vi "mqttCmdPublishAckCommand.vi"(9 "messageID":u16, 11 "error in (no error)":errorcluster) -> (15 "error out":errorcluster)   [LabVIEW 2015]
uses:
  mqttTypedef/mqttMessageType.ctl
  mqttTypedef/mqttQOSlevel.ctl
  mqttCmd.lvclass
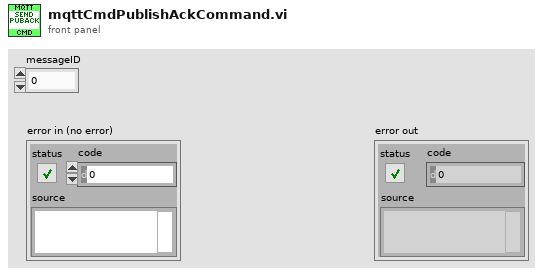
[diagram p1: front panel]
types:
  T1 = typedef "mqttQOSlevel.ctl" = enum8{"At most once", "At least once", "Exactly once", "Reserved"}
  T2 = typedef "mqttMessageType.ctl" = enum32{"Reserved", "CONNECT", "CONNACK", "PUBLISH", "PUBACK", "PUBREC", "PUBREL", "PUBCOMP", "SUBSCRIBE", "SUBACK", "UNSUBSCRIBE", "UNSUBACK", "PINGREQ", "PINGRESP", "DISCONNECT", "Reserved2"}
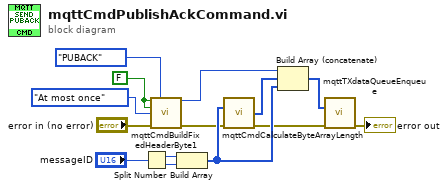
[diagram p0: block diagram]
diagram:
  w1 = FALSE ("retain(F)")
  n1 = Split Number(x="messageID") -> (hi(x)=w7:u8, lo(x)=w8:u8)
  n2 = call "mqttCmdBuildFixedHeaderByte1.vi"("retain(F)"=w1, "MessageType"=mqttMessageType."PUBACK", "duplicate(F)"=w1, "QoS (At most once)"=mqttQOSlevel."At most once", "error in (no error)"="error in (no error)") -> ("byte1"=w9:u8, "error out"=w4:errorcluster)  [unwired: 9 in]
  n3 = Build Array(w7, w8) -> (w5:u8[])
  n4 = call "mqttCmdCalculateByteArrayLength.vi"("byteArry in"=w5, "error in (no error)"=w4) -> ("length out"=w2:u8[], "error out"=w3:errorcluster)  [unwired: 12 in]
  n5 = Build Array (concatenate)(w9, w2, w5) -> (w10:u8[])
  n6 = call "mqttTXdataQueueEnqueue.vi"("data in"=w10, "error in (no error)"=w3) -> ("error out"=→"error out":errorcluster)  [unwired: 13 in]
